vi "Decimate array to lenght.vi"(8 "desired lenght":i32=8, 11 "Input array":sgl[](array[numeric])) -> (3 "Output array":sgl[](array[numeric]))   [LabVIEW 2021, in "MatS Libs.lvlib"]
doc: "Decimates array to givent lenght.\ndesired lenght has to be more or queal than 1 and less or equeal than size of array"
uses:
  <userlib>/MatS Libs/MatS Libs.lvlib
  <vilib>/GPower/Math/Library/Stat/Median/MedianSGL.vi
  <userlib>/_MGI/1D Array/MGI Average/MGI Average (SGL[]).vi
  <vilib>/GPower/Math/GPMath.lvlib
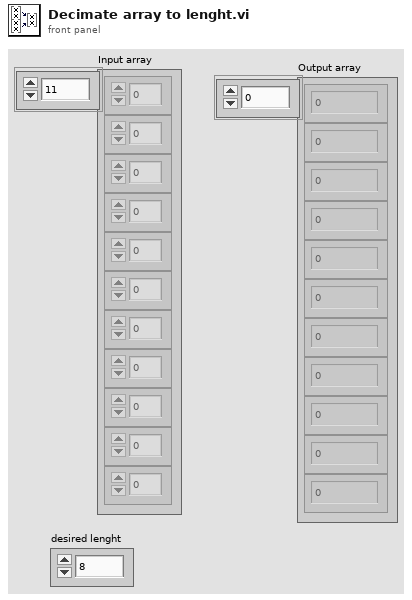
[diagram p1: front panel]
types:
  T1 = enum16{"Max", "Min", "Median", "Average", "First", "Last"}
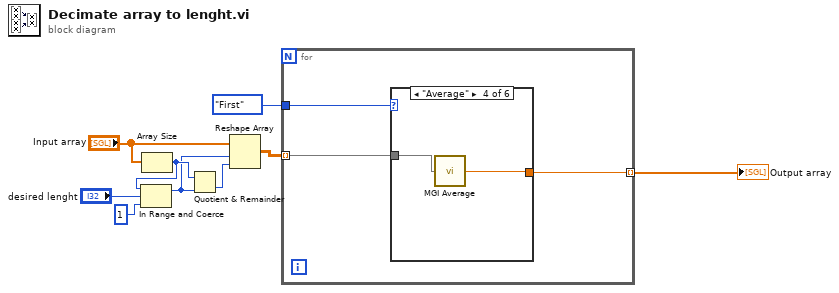
[diagram p0: block diagram]
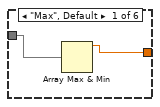
[diagram p2: hidden frame]
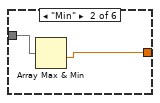
[diagram p3: hidden frame]
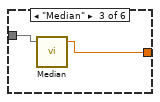
[diagram p4: hidden frame]
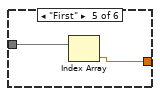
[diagram p5: hidden frame]
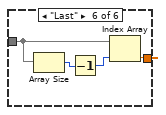
[diagram p6: hidden frame]
diagram:
  n1 = Array Size(array="Input array") -> (size(s)=w3:i32)
  n2 = In Range and Coerce(upper limit=w3, x="desired lenght", lower limit=1) -> (coerced(x)=w2:i32)  [unwired: 1 out]
  n3 = Quotient & Remainder(x=w3, y=w2) -> (floor(x/y)=w8:i32)  [unwired: 1 out]
  n4 = Reshape Array("Input array", w2, w8) -> (w9:sgl[][])
  n5 = for {
    tunnel: w9 -> [w12] mode=indexing
    tunnel: [w11] -> w7 mode=indexing
    tunnel: T1."First" ("Decimaion method") -> [w10]
    n6 = case shown="\"Average\"" w10 {
      tunnel: w12 -> [w14 w16 w18 w19 w22 w24]
      tunnel: [w13 w15 w17 w20 w21 w26] -> w11
      frame "Max", Default {
        n7 = Array Max & Min(array=w14) -> (max value=w13:sgl)  [unwired: 3 out]
      }
      frame "Min" {
        n8 = Array Max & Min(array=w16) -> (min value=w15:sgl)  [unwired: 3 out]
      }
      frame "Median" {
        n9 = call-poly <vilib>:"Median.vi"("X"=w18) -> ("Median"=w17:sgl)  [unwired: 4 in]
      }
      frame "Average" {
        n10 = call-poly <userlib>:"MGI Average.vi"("Single[]"=w19) -> ("Average"=w20:sgl)  [unwired: 1 in]
      }
      frame "First" {
        n11 = Index Array(array=w22) -> (element=w21:sgl)  [unwired: 1 in]
      }
      frame "Last" {
        n12 = Array Size(array=w24) -> (size(s)=w25:i32)
        n13 = Decrement(x=w25) -> (x-1=w23:i32)
        n14 = Index Array(array=w24, index=w23) -> (element=w26:sgl)
      }
    }
  }
  "Output array" <- w7
